vi "Rising Edge.vi"(1 "signal":bool) -> (0 "rising edge":bool)   [LabVIEW 2017, in "Communicable State Machine.lvlib"]
uses:
  Communicable State Machine.lvlib
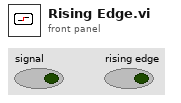
[diagram p1: front panel]
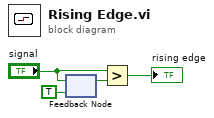
[diagram p0: block diagram]
diagram:
  n1 = feedback #1(TRUE) -> (w1:bool)
  n2 = feedback-in #1("signal") -> ()
  n3 = Greater?(x="signal", y=w1) -> (0:→"rising edge":bool)
